vi "Displacement Graph View.vi"(0 "Model in":refnum<class "Model.lvclass">) -> ()   [LabVIEW 2016, in "M1M3SupportEUI_Views.lvlib"]
uses:
  M1M3SupportEUI_Views.lvlib
  Typedefs/Display Displacement Types.ctl
  Model/Model.lvclass
  M1M3 Support Events/M1M3 Support Events.lvclass/M1M3 Support Events.ctl
  M1M3 Support Events/M1M3 Support Events.lvclass
  Typedefs/M1M3SupportEUI_TypeDefs.lvlib
panel:
  out "IMSRaw":T1 {"8" format="%.9f"; "7" format="%.9f"; "6" format="%.9f"; "4" format="%.9f"; "2" format="%.9f"; "5" format="%.9f"; "3" format="%.9f"; "1" format="%.9f"}
  out "IMS":T2 {"ZRotation" format="%.9f"; "YRotation" format="%.9f"; "XRotation" format="%.9f"; "ZPosition" format="%.9f"; "YPosition" format="%.9f"; "XPosition" format="%.9f"}
  out "Event Time Stamp":timestamp
  out "Unknown Problem":bool
  out "Unknown Command":bool
  out "Invalid Response":bool
  out "Invalid Length":bool
  out "Response Timeout":bool
  out "Write Control Error":bool
  out "Expansion Line Error":bool
  out "ID Number Error":bool
  out "Communication Error":bool
  out "Parameter Error":bool
  out "Number of Parameters Error":bool
  out "Data Length Error":bool
  out "Communication Timeout":bool
  out "Invalid Command":bool
  out "Any Warning":bool
  in  "Display Displacement Types":T3
  out "XY Graph":cluster{"Y":dbl[], "Y":dbl[]}[](graph)
  # "Position"
  # "Rotation"
  # "X"
  # "Y"
  # "Z"
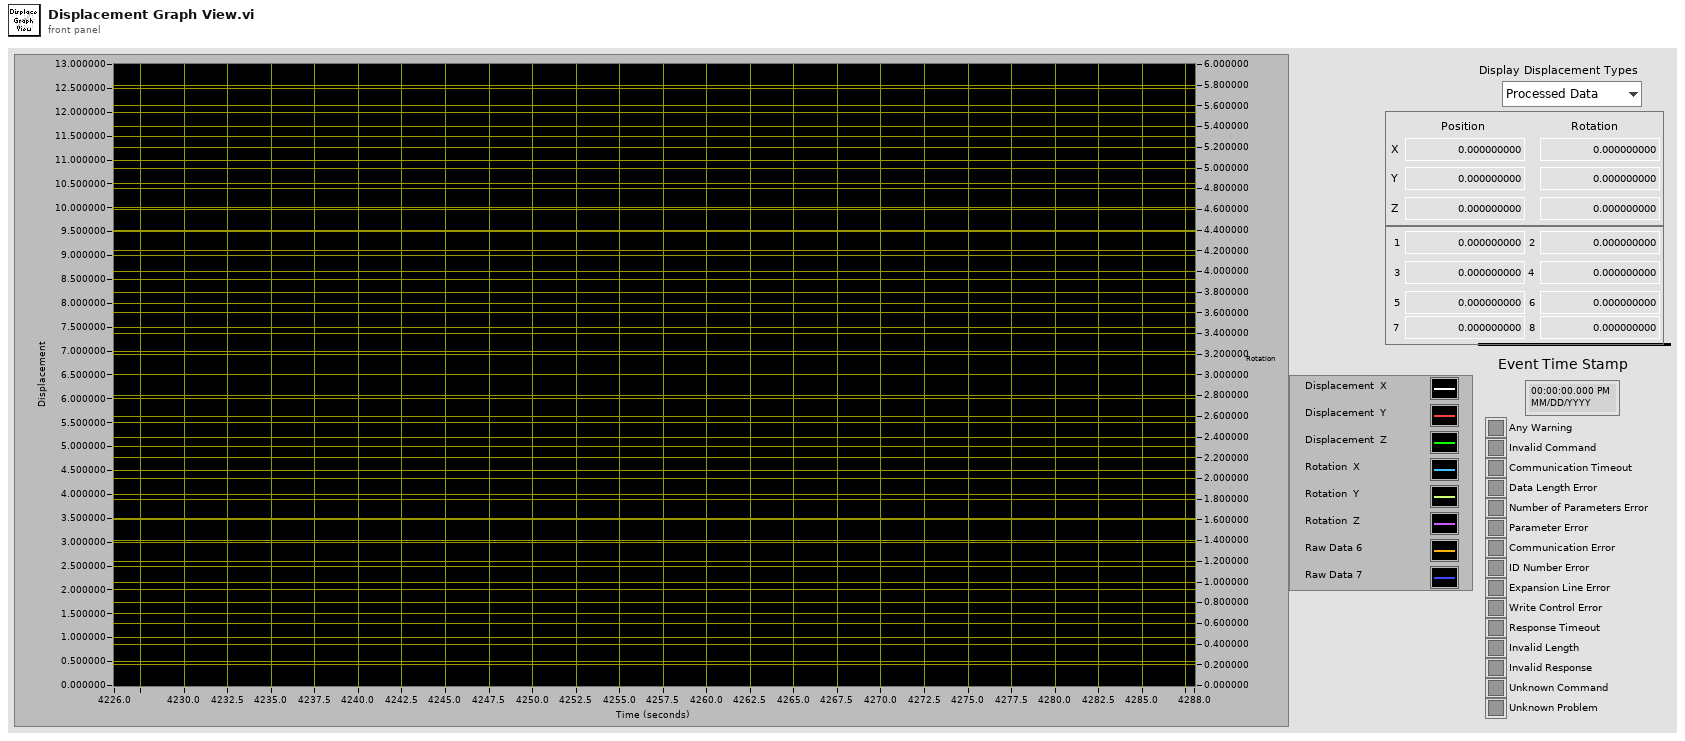
[diagram p1: front panel]
types:
  T1 = cluster{"1":dbl, "2":dbl, "3":dbl, "4":dbl, "5":dbl, "6":dbl, "7":dbl, "8":dbl}
  T2 = cluster{"XPosition":dbl, "YPosition":dbl, "ZPosition":dbl, "XRotation":dbl, "YRotation":dbl, "ZRotation":dbl}
  T3 = typedef "M1M3SupportEUI_TypeDefs.lvlib/Display Displacement Types.ctl" = enum16{"Processed Data", "Raw Data"}
  T4 = typedef "M1M3SupportEUI_TypeDefs.lvlib/M1M3 Support Events.ctl" = cluster{"Inclinometer  Data":refnum<user-event>, "IMS Data":refnum<user-event>, "SAL Connected":refnum<user-event>, "Accelerometer Data":refnum<user-event>, "OuterLoop Data":refnum<user-event>, "ErrorCode Event":refnum<user-event>, "InterlockStatus Event":refnum<user-event>, "InterlockWarning Event":refnum<user-event>, "Gyro Data":refnum<user-event>, "HP Actuator Info Event":refnum<user-event>, " FA Info Event":refnum<user-event>, "HP Monitor Info Event":refnum<user-event>, "FA Data":refnum<user-event>, "HP Actuator data":refnum<user-event>, "HP Monitor data":refnum<user-event>, "Air Supply Status Event":refnum<user-event>, "Air Supply Warning Event":refnum<user-event>, "Power Data":refnum<user-event>, "PID Data":refnum<user-event>, "PID Info Event":refnum<user-event>, "Power Status Event":refnum<user-event>, "Power Supply Status Event":refnum<user-event>, "Power Warning Event":refnum<user-event>, "Summary State Event":refnum<user-event>, "Detailed State Event":refnum<user-event>, "FA Force Warning Event":refnum<user-event>, "FA Warning Event":refnum<user-event>, "FA State Event":refnum<user-event>, "Applied AberrationForces Event":refnum<user-event>, "Applied Acceleration Forcces Event":refnum<user-event>, "Applied Azimuth Forces Event":refnum<user-event>, "Applied Active Optic Forces Event":refnum<user-event>, "Applied Balance Forces Event":refnum<user-event>, "Applied Cylinder Forces Event":refnum<user-event>, "Applied Elevation Forces Event":refnum<user-event>, "Applied Forces Event":refnum<user-event>, "Applied Offset Forces Event":refnum<user-event>, "Applied Static Forces Event":refnum<user-event>, "Applied Thermal Forces Event":refnum<user-event>, "Applied Velocity Forces Event":refnum<user-event>, "Rejected Aberration Force Event":refnum<user-event>, "Rejected Acceleration Forces Event":refnum<user-event>, "Rejected Active Optic Forces Event":refnum<user-event>, "Rejected Azimuth Forces Event":refnum<user-event>, "Rejected Balance Forces Event":refnum<user-event>, "Rejected Cylinder Forces Event":refnum<user-event>, "Rejected Elevation Forces Event":refnum<user-event>, "Rejected Forces Event":refnum<user-event>, "Rejected Offset Forces Event":refnum<user-event>, "Rejected Static Forces Event":refnum<user-event>, "Rejected Thermal Forces Event":refnum<user-event>, "Rejected Velocity Forces Event":refnum<user-event>, "Command Rejection Event":refnum<user-event>, "Setting Verions Event":refnum<user-event>, "Settings Applied Event":refnum<user-event>, "HP Actuator State Event":refnum<user-event>, "HP Actuator Warning Event":refnum<user-event>, "HP Monitor State Event":refnum<user-event>, "HP Monitor Warning Event":refnum<user-event>, "Accelerometer Warning Event":refnum<user-event>, "Applied Settings Match Start Event":refnum<user-event>, "Cell Light Status Event ":refnum<user-event>, "Cell Light Warning Event":refnum<user-event>, "Displacement Sensor Warning Event":refnum<user-event>, "Force Setpoint Warning Event":refnum<user-event>, "Gyro Warning Event ":refnum<user-event>, "ILC Warning Event ":refnum<user-event>, "Inclinometer Sensor Warning Event ":refnum<user-event>}
  T5 = enum16{"", "DetailedState_DetailedStates_DisabledState", "DetailedState_DetailedStates_EnabledState", "DetailedState_DetailedStates_FaultState", "DetailedState_DetailedStates_OfflineState", "DetailedState_DetailedStates_StandbyState", "DetailedState_DetailedStates_ParkedState", "DetailedState_DetailedStates_RaisingState", "DetailedState_DetailedStates_ActiveState", "DetailedState_DetailedStates_LoweringState", "DetailedState_DetailedStates_EngineeringState", "DetailedState_DetailedStates_ParkedEngineeringState", "DetailedState_DetailedStates_RaisingEngineeringState", "DetailedState_DetailedStates_ActiveEngineeringState", "DetailedState_DetailedStates_LoweringEngineeringState", "DetailedState_DetailedStates_LoweringFaultState", "DetailedState_DetailedStates_ProfileHardpointCorrectionState"}
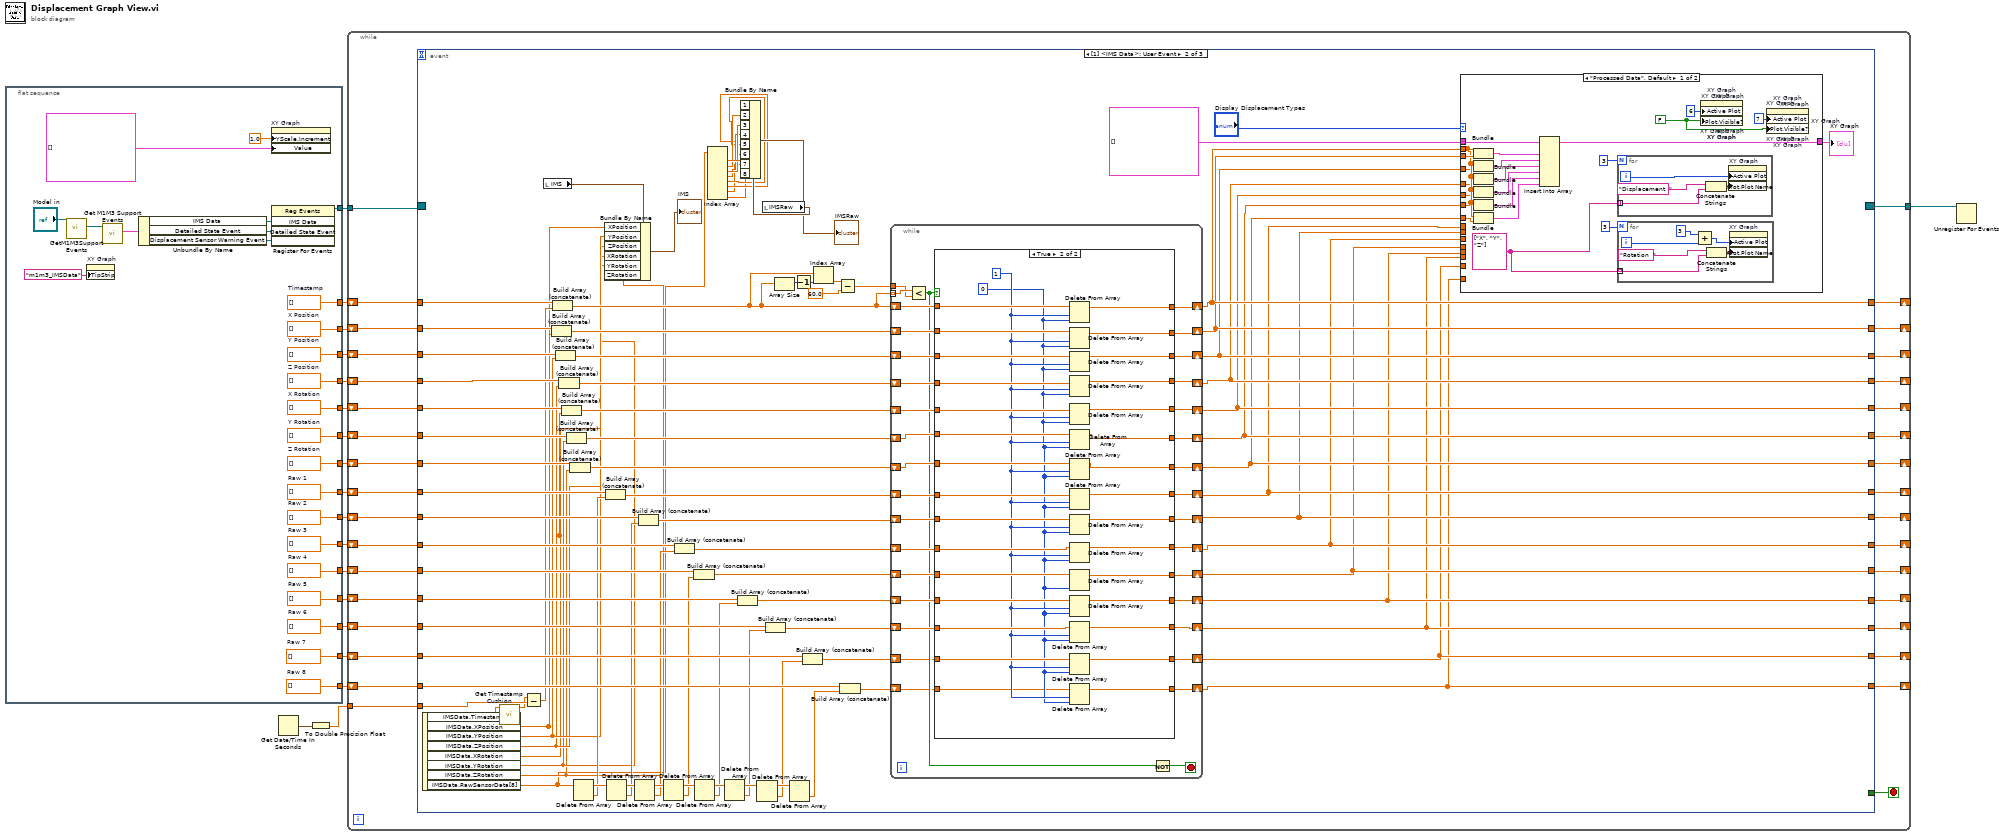
[diagram p0: block diagram]
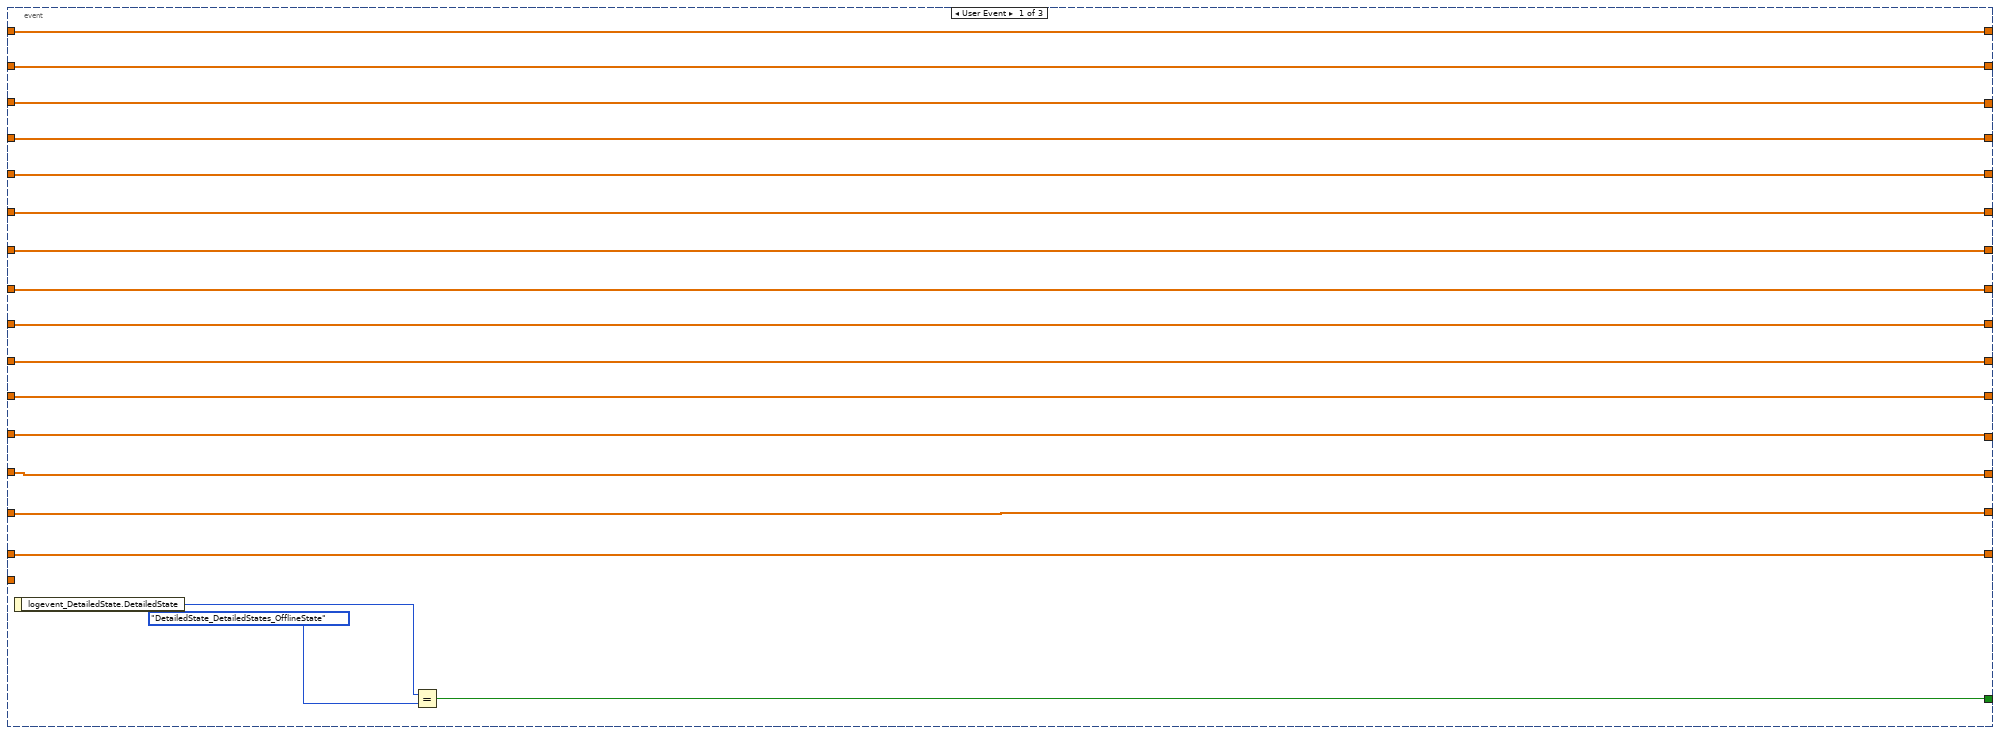
[diagram p2: hidden frame]
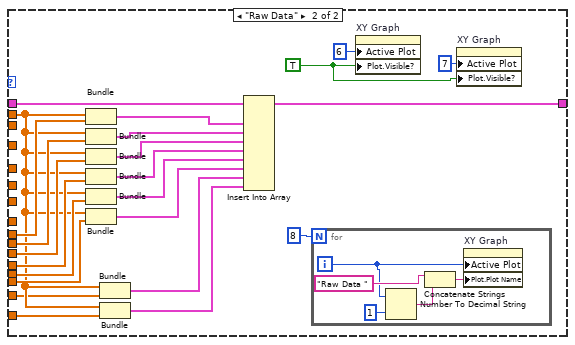
[diagram p4: hidden frame]
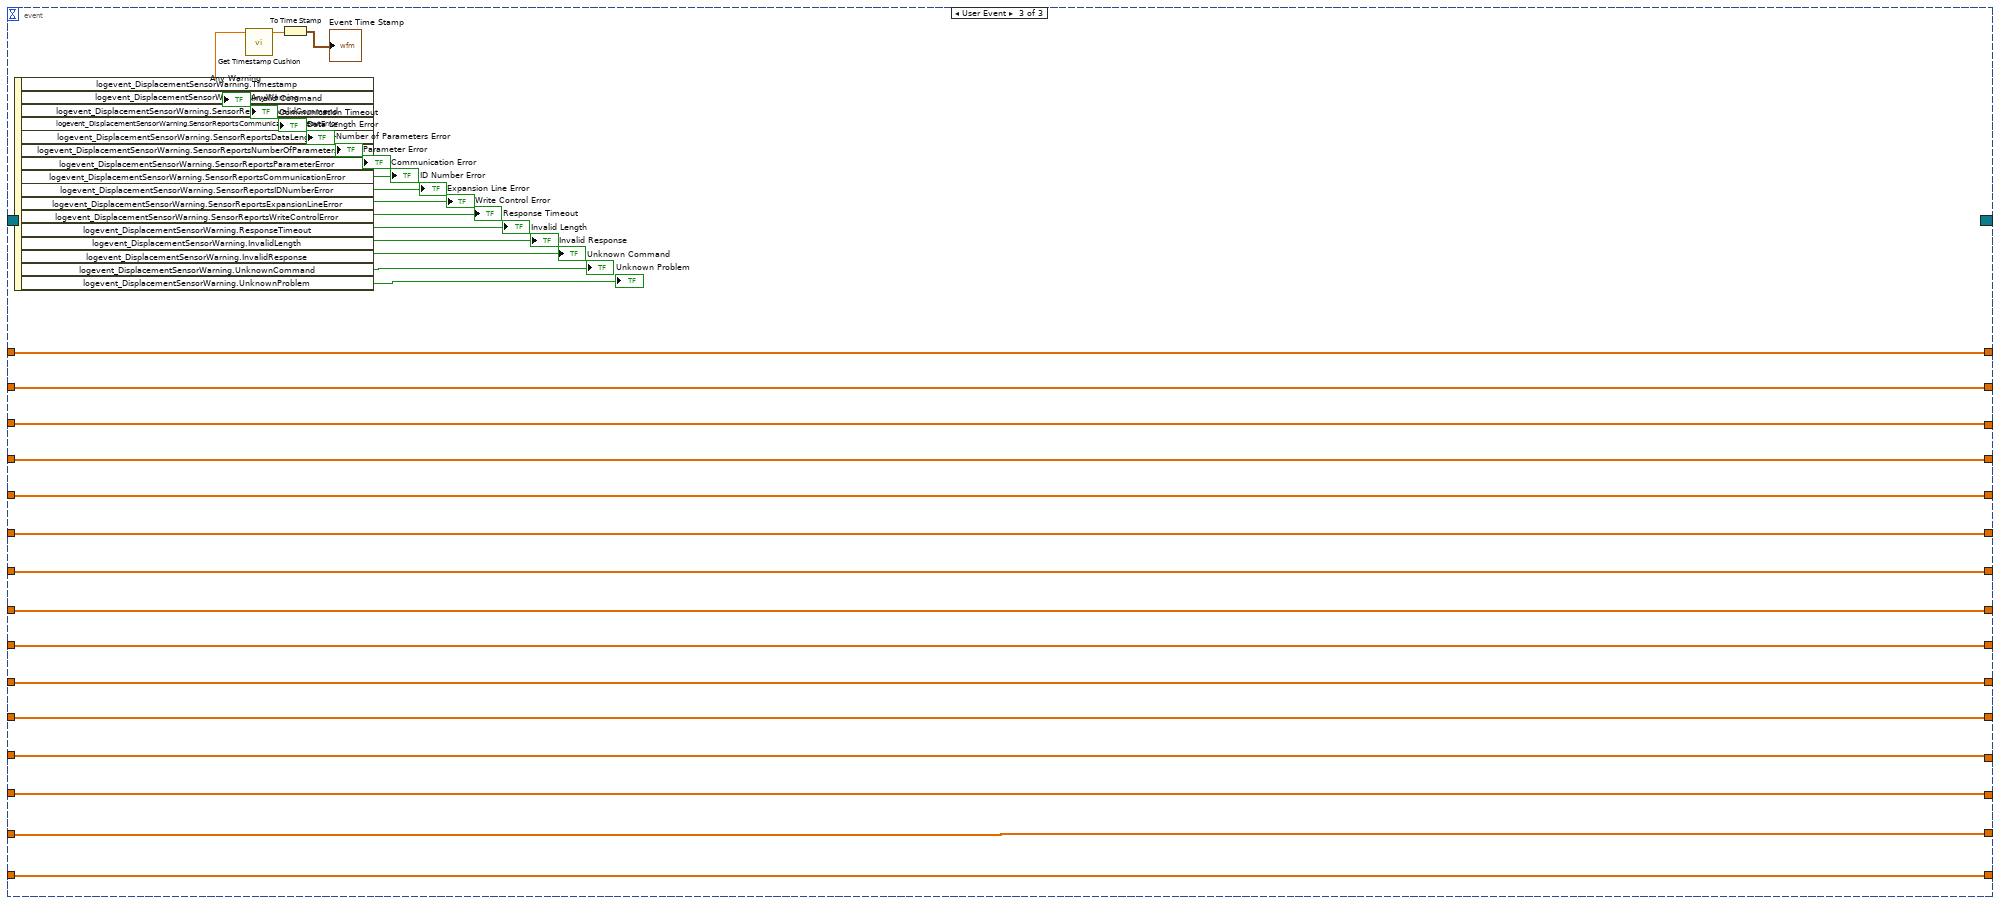
[diagram p5: hidden frame]
diagram:
  n1 = flat-sequence {
    tunnel: [w42] -> w19
    tunnel: [w41] -> w17
    tunnel: [w40] -> w16
    tunnel: [w39] -> w15
    tunnel: [w38] -> w14
    tunnel: [w37] -> w13
    tunnel: [w36] -> w12
    tunnel: [w35] -> w11
    tunnel: [w34] -> w10
    tunnel: [w33] -> w9
    tunnel: [w32] -> w8
    tunnel: [w31] -> w7
    tunnel: [w30] -> w6
    tunnel: [w29] -> w5
    tunnel: [w22] -> w4
    tunnel: [w21] -> w3
    frame #0 {
      w21 = sgl[] []  # Raw 8
      w22 = sgl[] []  # Raw 7
      w29 = sgl[] []  # Raw 6
      w30 = sgl[] []  # Raw 5
      w31 = sgl[] []  # Raw 4
      w32 = sgl[] []  # Raw 3
      w33 = sgl[] []  # Raw 2
      w34 = sgl[] []  # Raw 1
      w35 = sgl[] []  # Z Rotation
      w36 = sgl[] []  # Y Rotation
      w37 = sgl[] []  # X Rotation
      w38 = sgl[] []  # Z Position
      w39 = sgl[] []  # Y Position
      w40 = sgl[] []  # X Position
      w41 = dbl[] []  # Timestamp
      n2 = call "GetM1M3SupportEvents.vi"("Model in"="Model in") -> ("M1M3 Support Events out"=w24:refnum<class "M1M3 Support Events.lvclass">)  [unwired: 8 in, 2 out]
      n3 = property on="XY Graph" class="XYGraph (strict)"("TipStrip"="m1m3_IMSData" ("Tip Strip")) -> ()  [unwired: 2 in, 2 out]
      n4 = call "Get M1M3 Support Events.vi"("M1M3 Support Events in"=w24) -> ("M1M3 Support Events"=w43:T4)  [unwired: 9 in, 1 out]
      n5 = Unbundle By Name(w43) -> ("IMS Data"=w44:refnum<user-event>, "Detailed State Event"=w26:refnum<user-event>, "Displacement Sensor Warning Event"=w20:refnum<user-event>)
      n6 = property on="XY Graph" class="XYGraph (strict)"("YScale.Increment"=1.0 ("Y Scale.Range:Increment"), "Value"=cluster{dbl[], dbl[]}[] []) -> ()  [unwired: 2 in, 2 out]
      n7 = register-events(w44, w26, w20) -> (reference out=w42:refnum<event-registration>)  [unwired: 2 in, 1 out]
    }
  }
  n8 = Get Date/Time In Seconds() -> (seconds since 1Jan1904=w2:timestamp)
  n9 = To Double Precision Float(number=w2) -> (double precision float=w1:dbl)
  n10 = while {
    tunnel: w19 -> [w78]
    tunnel: [w76] -> w18
    shift-right: [w74] -> _
    shift-left: w17 -> [w75]
    shift-right: [w72] -> _
    shift-left: w16 -> [w73]
    shift-right: [w70] -> _
    shift-left: w15 -> [w71]
    shift-right: [w68] -> _
    shift-left: w14 -> [w69]
    shift-right: [w58] -> _
    shift-left: w13 -> [w67]
    shift-right: [w57] -> _
    shift-left: w12 -> [w66]
    shift-right: [w56] -> _
    shift-left: w11 -> [w65]
    shift-right: [w55] -> _
    shift-left: w10 -> [w64]
    shift-right: [w54] -> _
    shift-left: w9 -> [w63]
    shift-right: [w53] -> _
    shift-left: w8 -> [w62]
    shift-right: [w52] -> _
    shift-left: w7 -> [w61]
    shift-right: [w51] -> _
    shift-left: w6 -> [w60]
    shift-right: [w50] -> _
    shift-left: w5 -> [w59]
    shift-right: [w47] -> _
    shift-left: w4 -> [w49]
    shift-right: [w46] -> _
    shift-left: w3 -> [w48]
    tunnel: w1 -> [w45]
    stop <- w77 stop-if-true
    n11 = event shown="[1] <IMS Data>: User Event" {
      selector: w78 -> [_ _ _]
      dyn-events: [_ _ _] -> w76
      timeout: _ -> [_ _ _]
      tunnel: [w96 _ _] -> w77
      tunnel: w75 -> [w83 w187 w378]
      tunnel: [w83 w166 w378] -> w74
      tunnel: w73 -> [w84 w186 w377]
      tunnel: [w84 w164 w377] -> w72
      tunnel: w71 -> [w85 w185 w376]
      tunnel: [w85 w162 w376] -> w70
      tunnel: w69 -> [w86 w184 w375]
      tunnel: [w86 w160 w375] -> w68
      tunnel: w67 -> [w87 w183 w374]
      tunnel: w66 -> [w88 w182 w373]
      tunnel: w65 -> [w89 w181 w372]
      tunnel: w64 -> [w90 w180 w371]
      tunnel: w63 -> [w91 w178 w370]
      tunnel: w62 -> [w92 w176 w369]
      tunnel: w61 -> [w93 w174 w368]
      tunnel: w60 -> [w94 w172 w367]
      tunnel: w59 -> [w95 w170 w366]
      tunnel: [w87 w158 w374] -> w58
      tunnel: [w88 w156 w373] -> w57
      tunnel: [w89 w154 w372] -> w56
      tunnel: [w90 w152 w371] -> w55
      tunnel: [w91 w150 w370] -> w54
      tunnel: [w92 w148 w369] -> w53
      tunnel: [w93 w146 w368] -> w52
      tunnel: [w94 w144 w367] -> w51
      tunnel: [w95 w142 w366] -> w50
      tunnel: w49 -> [w79 w135 w365]
      tunnel: w48 -> [w80 w134 w364]
      tunnel: [w79 w129 w365] -> w47
      tunnel: [w80 w128 w364] -> w46
      tunnel: w45 -> [_ w117 _]
      event User Event {
        n12 = event-data() -> ("logevent_DetailedState.DetailedState"=w82:T5)  [unwired: 1 in]
        n13 = Equal?(x=w82, y=T5."DetailedState_DetailedStates_OfflineState") -> (x = y?=w96:bool)
      }
      event User Event {
        n14 = event-data() -> ("IMSData.Timestamp"=w118:dbl, "IMSData.XPosition"=w113:sgl, "IMSData.YPosition"=w112:sgl, "IMSData.ZPosition"=w111:sgl, "IMSData.XRotation"=w110:sgl, "IMSData.YRotation"=w109:sgl, "IMSData.ZRotation"=w108:sgl, "IMSData.RawSensorData[8]"=w105:sgl[])  [unwired: 1 in]
        n15 = call "Get Timestamp Cushion.vi"("DoubleTimestampRepresentation"=w118) -> ("TimestampCushion"=w116:dbl)  [unwired: 10 in]
        n16 = Subtract(x=w116, y=w117) -> (x-y=w119:dbl)
        n17 = local read "IMS"() -> (w114:T2)
        n18 = Build Array (concatenate)(w186, w113) -> (w165:sgl[])
        n19 = Build Array (concatenate)(w187, w119) -> (w136:dbl[])
        n20 = Build Array (concatenate)(w185, w112) -> (w163:sgl[])
        n21 = Build Array (concatenate)(w184, w111) -> (w161:sgl[])
        n22 = Build Array (concatenate)(w183, w110) -> (w159:sgl[])
        n23 = Build Array (concatenate)(w182, w109) -> (w157:sgl[])
        n24 = Build Array (concatenate)(w181, w108) -> (w155:sgl[])
        n25 = Delete From Array(array=w105) -> (deleted portion=w127:sgl, array with subset deleted=w179:sgl[])  [unwired: 2 in]
        n26 = Bundle By Name(cluster=w114, "XPosition"=w113, "YPosition"=w112, "ZPosition"=w111, "XRotation"=w110, "YRotation"=w109, "ZRotation"=w108) -> (→"IMS":T2)
        n27 = Build Array (concatenate)(w180, w127) -> (w153:sgl[])
        n28 = Delete From Array(array=w179) -> (deleted portion=w126:sgl, array with subset deleted=w177:sgl[])  [unwired: 2 in]
        n29 = Delete From Array(array=w177) -> (deleted portion=w125:sgl, array with subset deleted=w175:sgl[])  [unwired: 2 in]
        n30 = Build Array (concatenate)(w178, w126) -> (w151:sgl[])
        n31 = Delete From Array(array=w175) -> (deleted portion=w124:sgl, array with subset deleted=w173:sgl[])  [unwired: 2 in]
        n32 = Build Array (concatenate)(w176, w125) -> (w149:sgl[])
        n33 = Build Array (concatenate)(w174, w124) -> (w147:sgl[])
        n34 = Delete From Array(array=w173) -> (deleted portion=w123:sgl, array with subset deleted=w171:sgl[])  [unwired: 2 in]
        n35 = Index Array(array=w105) -> (element #1=w104:sgl, element #2=w103:sgl, element #3=w102:sgl, element #4=w101:sgl, element #5=w100:sgl, element #6=w99:sgl, element #7=w98:sgl, element #8=w97:sgl)  [unwired: 8 in]
        n36 = Delete From Array(array=w171) -> (deleted portion=w122:sgl, array with subset deleted=w133:sgl[])  [unwired: 2 in]
        n37 = Build Array (concatenate)(w172, w123) -> (w145:sgl[])
        n38 = Delete From Array(array=w133) -> (deleted portion=w121:sgl, array with subset deleted=w132:sgl[])  [unwired: 2 in]
        n39 = local read "IMSRaw"() -> (w107:T1)
        n40 = Bundle By Name(cluster=w107, "1"=w104, "2"=w103, "3"=w102, "4"=w101, "5"=w100, "6"=w99, "7"=w98, "8"=w97) -> (→"IMSRaw":T1)
        n41 = Build Array (concatenate)(w170, w122) -> (w143:sgl[])
        n42 = Array Size(array=w136) -> (size(s)=w139:i32)
        n43 = Delete From Array(array=w132) -> (deleted portion=w120:sgl)  [unwired: 2 in, 1 out]
        n44 = Decrement(x=w139) -> (x-1=w138:i32)
        n45 = Build Array (concatenate)(w135, w121) -> (w131:sgl[])
        n46 = Index Array(array=w136, index=w138) -> (element=w140:dbl)
        n47 = Subtract(x=w140, y=60.0) -> (x-y=w137:dbl)
        n48 = Build Array (concatenate)(w134, w120) -> (w130:sgl[])
        n49 = while {
          shift-right: [w218] -> w166
          shift-left: w136 -> [w219]
          shift-right: [w216] -> w164
          shift-left: w165 -> [w217]
          shift-right: [w214] -> w162
          shift-left: w163 -> [w215]
          shift-right: [w212] -> w160
          shift-left: w161 -> [w213]
          shift-right: [w210] -> w158
          shift-left: w159 -> [w211]
          shift-right: [w208] -> w156
          shift-left: w157 -> [w209]
          shift-right: [w206] -> w154
          shift-left: w155 -> [w207]
          shift-right: [w204] -> w152
          shift-left: w153 -> [w205]
          shift-right: [w202] -> w150
          shift-left: w151 -> [w203]
          shift-right: [w200] -> w148
          shift-left: w149 -> [w201]
          shift-right: [w198] -> w146
          shift-left: w147 -> [w199]
          shift-right: [w196] -> w144
          shift-left: w145 -> [w197]
          shift-right: [w194] -> w142
          shift-left: w143 -> [w195]
          tunnel: w137 -> [w220]
          tunnel: w136 -> [w221] mode=indexing
          shift-right: [w189] -> w129
          shift-left: w131 -> [w191]
          shift-right: [w188] -> w128
          shift-left: w130 -> [w190]
          stop <- w193 stop-if-true
          n50 = Less?(x=w221, y=w220) -> (x < y?=w192:bool)
          n51 = case shown="True" w192 {
            tunnel: w219 -> [w236 w268]
            tunnel: [w236 w267] -> w218
            tunnel: w217 -> [w235 w266]
            tunnel: [w235 w265] -> w216
            tunnel: w215 -> [w234 w264]
            tunnel: [w234 w263] -> w214
            tunnel: w213 -> [w233 w262]
            tunnel: [w233 w261] -> w212
            tunnel: w211 -> [w232 w260]
            tunnel: [w232 w259] -> w210
            tunnel: w209 -> [w231 w258]
            tunnel: [w231 w257] -> w208
            tunnel: w207 -> [w230 w256]
            tunnel: [w230 w255] -> w206
            tunnel: w205 -> [w229 w254]
            tunnel: [w229 w253] -> w204
            tunnel: w203 -> [w228 w252]
            tunnel: [w228 w251] -> w202
            tunnel: w201 -> [w227 w250]
            tunnel: [w227 w249] -> w200
            tunnel: w199 -> [w226 w248]
            tunnel: [w226 w247] -> w198
            tunnel: w197 -> [w225 w246]
            tunnel: [w225 w245] -> w196
            tunnel: w195 -> [w224 w244]
            tunnel: [w224 w243] -> w194
            tunnel: w191 -> [w223 w242]
            tunnel: w190 -> [w222 w239]
            tunnel: [w223 w238] -> w189
            tunnel: [w222 w237] -> w188
            frame False {
            }
            frame True {
              w241 = 1
              w240 = 0
              n52 = Delete From Array(array=w268, length=w241, index=w240) -> (array with subset deleted=w267:dbl[])  [unwired: 1 out]
              n53 = Delete From Array(array=w266, length=w241, index=w240) -> (array with subset deleted=w265:sgl[])  [unwired: 1 out]
              n54 = Delete From Array(array=w264, length=w241, index=w240) -> (array with subset deleted=w263:sgl[])  [unwired: 1 out]
              n55 = Delete From Array(array=w262, length=w241, index=w240) -> (array with subset deleted=w261:sgl[])  [unwired: 1 out]
              n56 = Delete From Array(array=w260, length=w241, index=w240) -> (array with subset deleted=w259:sgl[])  [unwired: 1 out]
              n57 = Delete From Array(array=w258, length=w241, index=w240) -> (array with subset deleted=w257:sgl[])  [unwired: 1 out]
              n58 = Delete From Array(array=w256, length=w241, index=w240) -> (array with subset deleted=w255:sgl[])  [unwired: 1 out]
              n59 = Delete From Array(array=w254, length=w241, index=w240) -> (array with subset deleted=w253:sgl[])  [unwired: 1 out]
              n60 = Delete From Array(array=w252, length=w241, index=w240) -> (array with subset deleted=w251:sgl[])  [unwired: 1 out]
              n61 = Delete From Array(array=w250, length=w241, index=w240) -> (array with subset deleted=w249:sgl[])  [unwired: 1 out]
              n62 = Delete From Array(array=w248, index=w240) -> (array with subset deleted=w247:sgl[])  [unwired: 1 in, 1 out]
              n63 = Delete From Array(array=w246, length=w241, index=w240) -> (array with subset deleted=w245:sgl[])  [unwired: 1 out]
              n64 = Delete From Array(array=w244, length=w241, index=w240) -> (array with subset deleted=w243:sgl[])  [unwired: 1 out]
              n65 = Delete From Array(array=w242, length=w241, index=w240) -> (array with subset deleted=w238:sgl[])  [unwired: 1 out]
              n66 = Delete From Array(array=w239, length=w241, index=w240) -> (array with subset deleted=w237:sgl[])  [unwired: 1 out]
            }
          }
          n67 = Not(x=w192) -> (.not. x?=w193:bool)
        }
        n68 = case shown="\"Processed Data\", Default" "Display Displacement Types" {
          tunnel: w166 -> [w304 w325]
          tunnel: w164 -> [w307 _]
          tunnel: cluster{dbl[], dbl[]}[] [] -> [w306 w335]
          tunnel: w162 -> [w303 _]
          tunnel: w160 -> [w302 _]
          tunnel: w158 -> [w301 _]
          tunnel: w156 -> [w299 _]
          tunnel: w154 -> [w298 _]
          tunnel: [w293 w328] -> w167
          tunnel: w152 -> [_ w334]
          tunnel: w150 -> [_ w329]
          tunnel: w148 -> [_ w330]
          tunnel: w146 -> [_ w331]
          tunnel: w144 -> [_ w332]
          tunnel: w142 -> [_ w333]
          tunnel: w129 -> [_ w324]
          tunnel: w128 -> [_ w323]
          frame "Processed Data", Default {
            w269 = FALSE ("Plot.Visible")
            w274 = FALSE ("Plot.Visible")
            w277 = FALSE ("Plot.Visible")
            w280 = FALSE ("Plot.Visible")
            w281 = FALSE ("Plot.Visible")
            w286 = FALSE ("Plot.Visible")
            w287 = FALSE ("Plot.Visible")
            w290 = string[] ["X", "Y", "Z"]
            n69 = Bundle(w304, w307) -> (w305:cluster{dbl[], sgl[]})  [unwired: 1 in]
            n70 = Bundle(w304, w303) -> (w300:cluster{dbl[], sgl[]})  [unwired: 1 in]
            n71 = Bundle(w304, w302) -> (w294:cluster{dbl[], sgl[]})  [unwired: 1 in]
            n72 = Bundle(w304, w301) -> (w295:cluster{dbl[], sgl[]})  [unwired: 1 in]
            n73 = Bundle(w304, w299) -> (w296:cluster{dbl[], sgl[]})  [unwired: 1 in]
            n74 = Bundle(w304, w298) -> (w297:cluster{dbl[], sgl[]})  [unwired: 1 in]
            n75 = Insert Into Array(array=w306, new element #1=w305, new element #2=w300, new element #3=w294, new element #4=w295, new element #5=w296, new element #6=w297) -> (w293:cluster{dbl[], dbl[]}[])  [unwired: 1 in]
            n76 = for {
              N: 3 -> [_]
              tunnel: w290 -> [w314] mode=indexing
              i -> [w315]
              n77 = Concatenate Strings("Displacement  ", w314) -> (w317:string)
              n78 = property on="XY Graph" class="XYGraph (strict)"("Active Plot"=w315, "Plot.Plot Name"=w317) -> ()  [unwired: 2 in, 2 out]
            }
            n79 = for {
              N: 3 -> [_]
              tunnel: w290 -> [w308] mode=indexing
              i -> [w310]
              n80 = Add(x=3, y=w310) -> (x+y=w309:i32)
              n81 = Concatenate Strings("Rotation  ", w308) -> (w313:string)
              n82 = property on="XY Graph" class="XYGraph (strict)"("Active Plot"=w309, "Plot.Plot Name"=w313) -> ()  [unwired: 2 in, 2 out]
            }
            n83 = property on="XY Graph" class="XYGraph (strict)"("Active Plot"=u32 6, "Plot.Visible?"=w269) -> ()  [unwired: 2 in, 2 out]
            n84 = property on="XY Graph" class="XYGraph (strict)"("Active Plot"=u32 6, "Plot.Visible?"=w274) -> ()  [unwired: 2 in, 2 out]
            n85 = property on="XY Graph" class="XYGraph (strict)"("Active Plot"=u32 6, "Plot.Visible?"=w277) -> ()  [unwired: 2 in, 2 out]
            n86 = property on="XY Graph" class="XYGraph (strict)"("Active Plot"=u32 6, "Plot.Visible?"=w280) -> ()  [unwired: 2 in, 2 out]
            n87 = property on="XY Graph" class="XYGraph (strict)"("Active Plot"=u32 6, "Plot.Visible?"=w281) -> ()  [unwired: 2 in, 2 out]
            n88 = property on="XY Graph" class="XYGraph (strict)"("Active Plot"=u32 6, "Plot.Visible?"=w286) -> ()  [unwired: 2 in, 2 out]
            n89 = property on="XY Graph" class="XYGraph (strict)"("Active Plot"=u32 6, "Plot.Visible?"=w287) -> ()  [unwired: 2 in, 2 out]
            n90 = property on="XY Graph" class="XYGraph (strict)"("Active Plot"=u32 7, "Plot.Visible?"=w269) -> ()  [unwired: 2 in, 2 out]
            n91 = property on="XY Graph" class="XYGraph (strict)"("Active Plot"=u32 7, "Plot.Visible?"=w274) -> ()  [unwired: 2 in, 2 out]
            n92 = property on="XY Graph" class="XYGraph (strict)"("Active Plot"=u32 7, "Plot.Visible?"=w277) -> ()  [unwired: 2 in, 2 out]
            n93 = property on="XY Graph" class="XYGraph (strict)"("Active Plot"=u32 7, "Plot.Visible?"=w280) -> ()  [unwired: 2 in, 2 out]
            n94 = property on="XY Graph" class="XYGraph (strict)"("Active Plot"=u32 7, "Plot.Visible?"=w281) -> ()  [unwired: 2 in, 2 out]
            n95 = property on="XY Graph" class="XYGraph (strict)"("Active Plot"=u32 7, "Plot.Visible?"=w286) -> ()  [unwired: 2 in, 2 out]
            n96 = property on="XY Graph" class="XYGraph (strict)"("Active Plot"=u32 7, "Plot.Visible?"=w287) -> ()  [unwired: 2 in, 2 out]
          }
          frame "Raw Data" {
            w318 = TRUE ("Plot.Visible")
            n97 = Bundle(w325, w334) -> (w340:cluster{dbl[], sgl[]})  [unwired: 1 in]
            n98 = Bundle(w325, w329) -> (w339:cluster{dbl[], sgl[]})  [unwired: 1 in]
            n99 = Bundle(w325, w330) -> (w336:cluster{dbl[], sgl[]})  [unwired: 1 in]
            n100 = Bundle(w325, w331) -> (w337:cluster{dbl[], sgl[]})  [unwired: 1 in]
            n101 = Bundle(w325, w332) -> (w338:cluster{dbl[], sgl[]})  [unwired: 1 in]
            n102 = Bundle(w325, w333) -> (w326:cluster{dbl[], sgl[]})  [unwired: 1 in]
            n103 = Bundle(w325, w324) -> (w321:cluster{dbl[], sgl[]})  [unwired: 1 in]
            n104 = Bundle(w325, w323) -> (w322:cluster{dbl[], sgl[]})  [unwired: 1 in]
            n105 = Insert Into Array(array=w335, new element #1=w340, new element #2=w339, new element #3=w336, new element #4=w337, new element #5=w338, new element #6=w326, new element #7=w321, new element #8=w322) -> (w328:cluster{dbl[], dbl[]}[])  [unwired: 1 in]
            n106 = for {
              N: 8 -> [_]
              i -> [w342]
              n107 = Number To Decimal String(number=w342, width (-)=i16 1) -> (decimal integer string=w343:string)
              n108 = Concatenate Strings("Raw Data ", w343) -> (w345:string)
              n109 = property on="XY Graph" class="XYGraph (strict)"("Active Plot"=w342, "Plot.Plot Name"=w345) -> ()  [unwired: 2 in, 2 out]
            }
            n110 = property on="XY Graph" class="XYGraph (strict)"("Active Plot"=u32 6, "Plot.Visible?"=w318) -> ()  [unwired: 2 in, 2 out]
            n111 = property on="XY Graph" class="XYGraph (strict)"("Active Plot"=u32 7, "Plot.Visible?"=w318) -> ()  [unwired: 2 in, 2 out]
          }
        }
        "XY Graph" <- w167
      }
      event User Event {
        n112 = event-data() -> ("logevent_DisplacementSensorWarning.Timestamp"=w362:dbl, "logevent_DisplacementSensorWarning.AnyWarning"=→"Any Warning":bool, "logevent_DisplacementSensorWarning.SensorReportsInvalidCommand"=→"Invalid Command":bool, "logevent_DisplacementSensorWarning.SensorReportsCommunicationTimeoutError"=→"Communication Timeout":bool, "logevent_DisplacementSensorWarning.SensorReportsDataLengthError"=→"Data Length Error":bool, "logevent_DisplacementSensorWarning.SensorReportsNumberOfParametersError"=→"Number of Parameters Error":bool, "logevent_DisplacementSensorWarning.SensorReportsParameterError"=→"Parameter Error":bool, "logevent_DisplacementSensorWarning.SensorReportsCommunicationError"=→"Communication Error":bool, "logevent_DisplacementSensorWarning.SensorReportsIDNumberError"=→"ID Number Error":bool, "logevent_DisplacementSensorWarning.SensorReportsExpansionLineError"=→"Expansion Line Error":bool, "logevent_DisplacementSensorWarning.SensorReportsWriteControlError"=→"Write Control Error":bool, "logevent_DisplacementSensorWarning.ResponseTimeout"=→"Response Timeout":bool, "logevent_DisplacementSensorWarning.InvalidLength"=→"Invalid Length":bool, "logevent_DisplacementSensorWarning.InvalidResponse"=→"Invalid Response":bool, "logevent_DisplacementSensorWarning.UnknownCommand"=→"Unknown Command":bool, "logevent_DisplacementSensorWarning.UnknownProblem"=→"Unknown Problem":bool)  [unwired: 1 in]
        n113 = call "Get Timestamp Cushion.vi"("DoubleTimestampRepresentation"=w362) -> ("TimestampCushion"=w363:dbl)  [unwired: 10 in]
        n114 = To Time Stamp(1:w363) -> (0:→"Event Time Stamp":timestamp)
      }
    }
  }
  n115 = Unregister For Events(event registration refnum=w18) -> ()  [unwired: 1 in, 1 out]
